vi "Global.vi"() -> ()   [LabVIEW 2013]
uses:
  Model.ctl
  ParaConfig.ctl
panel:
  in  "参数配置":T1
  in  "设备型号AB":T2
  in  "MainPath":path
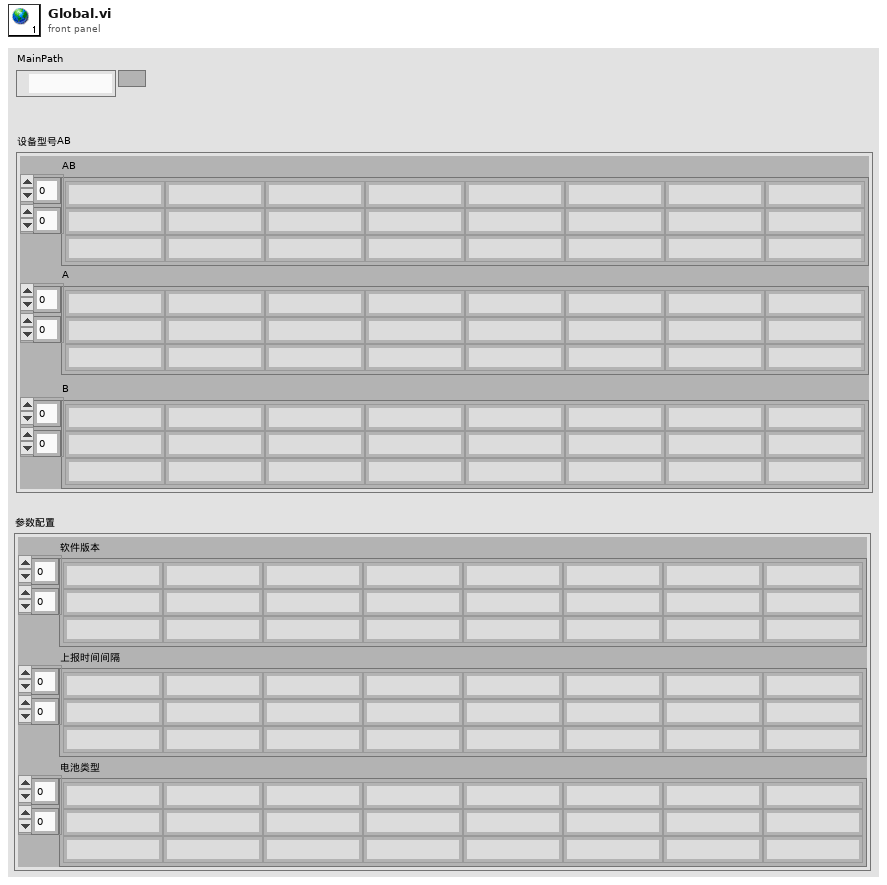
[diagram p1: front panel]
types:
  T1 = typedef "ParaConfig.ctl" = cluster{"软件版本":string[][], "上报时间间隔":string[][], "电池类型":string[][]}
  T2 = typedef "Model.ctl" = cluster{"AB":string[][], "A":string[][], "B":string[][]}
diagram:
